vi "Fix and Inline Core.vi"(7 "Just Fixup":bool, 8 "error in (no error)":errorcluster, 10 "SubVI Refnum in":refnum<vi>, 11 "VI in":refnum<vi>) -> (0 "error out":errorcluster)   [LabVIEW 2020, in "vim-liner.lvlib"]
uses:
  vim-liner.lvlib
  885a5e10-50e1-4279-8097-7d5ae3475e26.vi
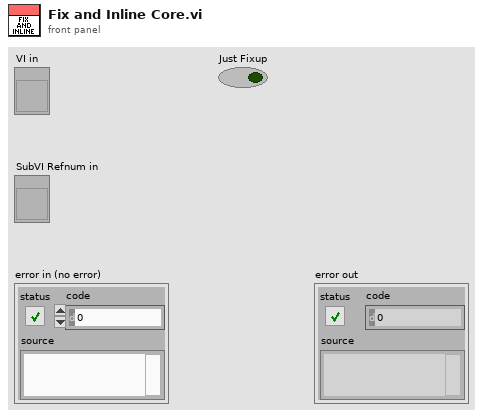
[diagram p1: front panel]
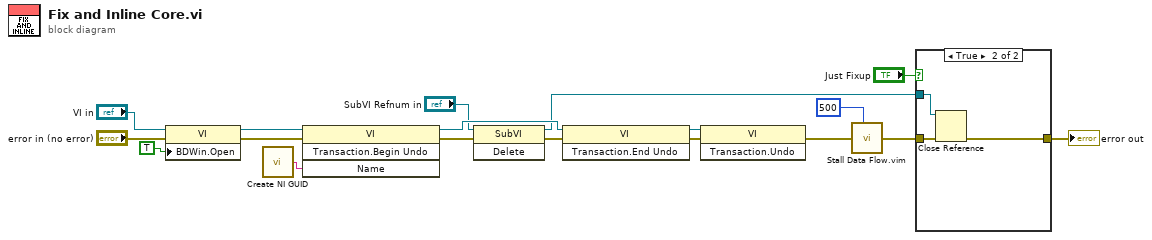
[diagram p0: block diagram]
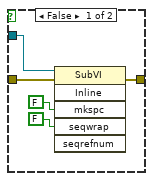
[diagram p2: hidden frame]
diagram:
  n1 = property class="VI"(reference="VI in", error in="error in (no error)", "BDWin.Open"=TRUE ("Block Diagram Window:Open")) -> (reference out=w11:refnum<vi>, error out=w9:errorcluster)
  n2 = call <vilib>:"Create NI GUID.vi"() -> ("NI GUID"=w18:string)
  n3 = invoke class="VI" method="Transaction.Begin Undo"(reference=w11, error in=w9, "Name"=w18) -> (reference out=w15:refnum<vi>, error out=w17:errorcluster)  [unwired: 1 in, 2 out]
  n4 = invoke class="SubVI" method="Delete"(reference="SubVI Refnum in", error in=w17) -> (reference out=w5:refnum<vi>, error out=w16:errorcluster)  [unwired: 1 in, 1 out]
  n5 = invoke class="VI" method="Transaction.End Undo"(reference=w15, error in=w16) -> (reference out=w14:refnum<vi>, error out=w13:errorcluster)  [unwired: 1 in, 1 out]
  n6 = invoke class="VI" method="Transaction.Undo"(reference=w14, error in=w13) -> (error out=w12:errorcluster)  [unwired: 1 in, 2 out]
  n7 = call "Stall Data Flow.vim"("value in"=w12, "milliseconds to wait"=u32 500) -> ("value out"=w3:errorcluster)  [unwired: 1 out]
  n8 = case shown="True" "Just Fixup" {
    tunnel: w5 -> [w23 w26]
    tunnel: [w22 w24] -> w1
    tunnel: w3 -> [w21 w25]
    frame False {
      n9 = invoke class="SubVI" method="Inline"(reference=w23, error in=w21, "mkspc"=FALSE ("Make Space in Block Diagram"), "seqwrap"=FALSE ("Wrap in Sequence")) -> (error out=w22:errorcluster)  [unwired: 2 in, 5 out]
    }
    frame True {
      n10 = Close Reference(reference=w26, error in (no error)=w25) -> (error out=w24:errorcluster)
    }
  }
  "error out" <- w1
